vi "Configure Parallel Execution.vi"(8 "error in (no error)":errorcluster, 9 "Persist?":bool, 10 "Enable Parallel Execution?":bool, 11 "Execution UI In":refnum<class "Execution UI.lvclass">) -> (0 "error out":errorcluster, 3 "Execution UI Out":refnum<class "Execution UI.lvclass">)   [LabVIEW 2020, in "Execution UI.lvclass"]
uses:
  Execution UI.lvclass
  C:/git/astemes-lunit/source/Framework/Result Observer/Result Observer.lvclass
  Execution UI.lvclass/Execution UI.ctl
  Framework/Single Thread Test Runner/Single Thread Test Runner.lvclass
  C:/git/astemes-lunit/source/Framework/Test Runner/Test Runner.lvclass
  Framework/Parallell Test Runner/Parallell Test Runner.lvclass
  <vilib>/Utility/sysdir.llb/Get System Directory.vi
  <vilib>/Utility/libraryn.llb/Create Directory Recursive.vi
  Framework/Test Runner/Test Runner.lvclass
  Configuration Manager/Configuration Manager.lvclass
  Support/Paths.lvlib
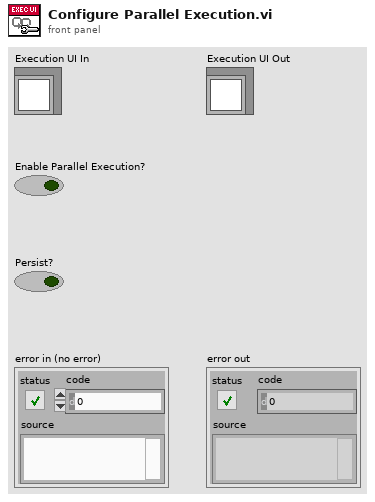
[diagram p1: front panel]
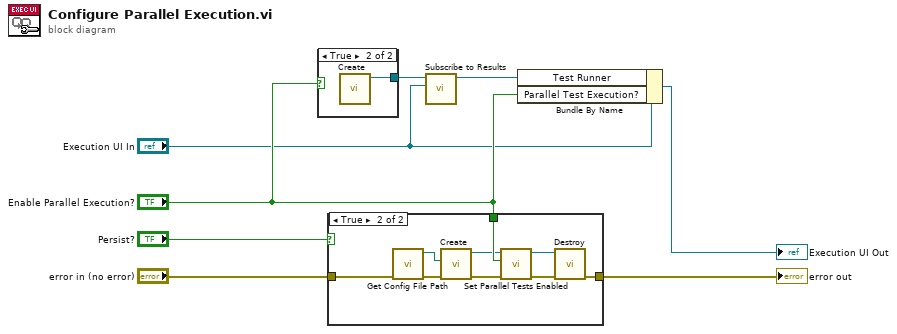
[diagram p0: block diagram]
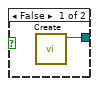
[diagram p3: hidden frame]
diagram:
  n1 = case shown="True" "Enable Parallel Execution?" {
    tunnel: [w9 w10] -> w5
    frame False {
      n2 = call "Create.vi"() -> ("Single Thread Test Runner out"=w9:refnum<class "Single Thread Test Runner.lvclass">)  [unwired: 10 in, 1 out]
    }
    frame True {
      n3 = call "Create.vi"() -> ("Parallell Test Runner out"=w10:refnum<class "Parallell Test Runner.lvclass">)  [unwired: 10 in, 1 out]
    }
  }
  n4 = case shown="True" "Persist?" {
    tunnel: "Enable Parallel Execution?" -> [_ w20]
    tunnel: [w11 w17] -> w4
    tunnel: "error in (no error)" -> [w11 w16]
    frame False {
    }
    frame True {
      n5 = call "Get Config File Path.vi"("error in (no error)"=w16) -> ("error out"=w14:errorcluster, "Config Directory"=w15:path)  [unwired: 9 in]
      n6 = call "Create.vi"("error in (no error)"=w14, "configuration file path"=w15) -> ("error out"=w19:errorcluster, "Configuration Manager out"=w18:refnum<class "Configuration Manager.lvclass">)  [unwired: 8 in]
      n7 = call "Set Parallel Tests Enabled.vi"("error in (no error)"=w19, "Parallel tests enabled?"=w20, "Configuration Manager In"=w18) -> ("error out"=w13:errorcluster, "Configuration Manager Out"=w12:refnum<class "Configuration Manager.lvclass">)  [unwired: 7 in]
      n8 = call "Destroy.vi"("error in (no error)"=w13, "Configuration Manager In"=w12) -> ("error out"=w17:errorcluster)  [unwired: 9 in]
    }
  }
  "error out" <- w4
  n9 = call-dynamic "Subscribe to Results.vi"("Result Observer"="Execution UI In", "Test Runner In"=w5) -> ("Test Runner Out"=w7:refnum<class "Test Runner.lvclass">)  [unwired: 8 in, 1 out]
  n10 = Bundle By Name(cluster="Execution UI In", "Test Runner"=w7, "Parallel Test Execution?"="Enable Parallel Execution?") -> (→"Execution UI Out":refnum<class "Execution UI.lvclass">)
